vi "PIM Stimulus Key Array.vi"(4 "Conversion":enum16{"Cluster - HTML", "HTML - Cluster"}(ring), 6 "PIM Test Parameters":T1={"Stimulus"={"C1 Pwr dBm"=0.0, "C2 Pwr dBm"=0.0, "Power Units"=enum."dBm", "Meas Type"=enum."Time", "C1 Freq MHz"=0.0, "C2 Freq MHz"=0.0, "Swept Freq Step"=0}, "Measure"={"IM Order"=0, "Direction"=0, "Averaging"=1, "ALC ON?"=TRUE, "Peak Hold?"=TRUE, "Peak last N"=1, "Ref Level dBm"=-100.0, "Ref Units"=enum."dBm", "Num Samples"=1, "Sample units"=enum."Sample(s)", "Update Rate (s)"=0.0, "DUT PORT"=enum."Port 1", "Percent (%)"=100}, "Display"={"Power Scale"={"yRange_min"=0, "yRange_max"=0}, "xRange_span"=5}} {"Stimulus"."Swept Freq Step" items=[".2", ".4", "1.0", "2.0"]; "Measure"."Averaging" items=["None", "Minimum", "Normal", "High", "Maximum"]; "Measure"."Direction" items=["Reverse", "Forward", "Auxiliary"]; "Measure"."IM Order" items=["3rd", "5th", "7th", "9th", "11th", "13th", "15th", "17th", "19th", "21st", "23rd", "25th", "27th", "29th", "31st", "33rd"]}, 7 "Key Array In":T11) -> (1 "PIM Test Parameters (out)":T1={"Stimulus"={"C1 Pwr dBm"=0.0, "C2 Pwr dBm"=0.0, "Power Units"=enum."dBm", "Meas Type"=enum."Time", "C1 Freq MHz"=0.0, "C2 Freq MHz"=0.0, "Swept Freq Step"=0}, "Measure"={"IM Order"=0, "Direction"=0, "Averaging"=1, "ALC ON?"=TRUE, "Peak Hold?"=TRUE, "Peak last N"=1, "Ref Level dBm"=-100.0, "Ref Units"=enum."dBm", "Num Samples"=1, "Sample units"=enum."Sample(s)", "Update Rate (s)"=0.0, "DUT PORT"=enum."Port 1", "Percent (%)"=100}, "Display"={"Power Scale"={"yRange_min"=0, "yRange_max"=0}, "xRange_span"=5}} {"Stimulus"."Swept Freq Step" items=[".2", ".4", "1.0", "2.0"]; "Measure"."Averaging" items=["None", "Minimum", "Normal", "High", "Maximum"]; "Measure"."Direction" items=["Reverse", "Forward", "Auxiliary"]; "Measure"."IM Order" items=["3rd", "5th", "7th", "9th", "11th", "13th", "15th", "17th", "19th", "21st", "23rd", "25th", "27th", "29th", "31st", "33rd"]}, 2 "Key Array Out":T11)   [LabVIEW 2011]
uses:
  ITK/utils/keyedarr.llb/Keyed Array.ctl
  TypeDefs/PIM Test Parameters.ctl
  TypeDefs/PIM Stimulus Parameters.ctl
  BPIMCore/HW IO/PIM Sweep Step Size.ctl
  TypeDefs/PIM Measurement Parameters.ctl
  BPIMCore/HW IO/IMOrder.ctl
  BPIMCore/HW IO/MeasMode.ctl
  BPIMCore/HW IO/HW Averaging.ctl
  TypeDefs/PIM Meas Units.ctl
  BPIMCore/HW IO/DUTport.ctl
  TypeDefs/PIM Display Parameters.ctl
  ITK/utils/strutil.llb/Case Matching.ctl
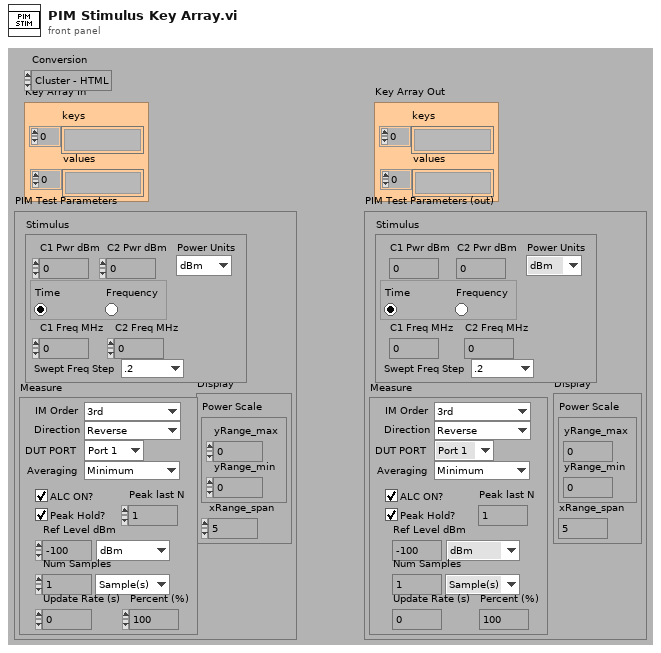
[diagram p1: front panel]
types:
  T1 = typedef "PIM Test Parameters.ctl" = cluster{"Stimulus":T2, "Measure":T4, "Display":T10}
  T2 = typedef "PIM Stimulus Parameters.ctl" = cluster{"C1 Pwr dBm":dbl, "C2 Pwr dBm":dbl, "Power Units":enum16{"dBm", "Watts"}, "Meas Type":enum32{"Time", "Frequency"}, "C1 Freq MHz":dbl, "C2 Freq MHz":dbl, "Swept Freq Step":T3}
  T3 = typedef "PIM Sweep Step Size.ctl" = u16
  T4 = typedef "PIM Measurement Parameters.ctl" = cluster{"IM Order":T5, "Direction":T6, "Averaging":T7, "ALC ON?":bool, "Peak Hold?":bool, "Peak last N":u32, "Ref Level dBm":dbl, "Ref Units":enum16{"dBm", "dBc"}, "Num Samples":u32, "Sample units":T8, "Update Rate (s)":dbl, "DUT PORT":T9, "Percent (%)":u8}
  T5 = typedef "IMOrder.ctl" = u8
  T6 = typedef "MeasMode.ctl" = u16
  T7 = typedef "HW Averaging.ctl" = u16
  T8 = typedef "PIM Meas Units.ctl" = enum16{"Sample(s)", "Second(s)", "Sweep(s)"}
  T9 = typedef "DUTport.ctl" = enum16{"Port 1", "Port 2"}
  T10 = typedef "PIM Display Parameters.ctl" = cluster{"Power Scale":cluster{"yRange_min":i32, "yRange_max":i32}, "xRange_span":u32}
  T11 = typedef "Keyed Array.ctl" = cluster{"keys":string[], "values":string[]}
  T12 = typedef "Case Matching.ctl" = enum16{"a != A", "a == A", "system"}
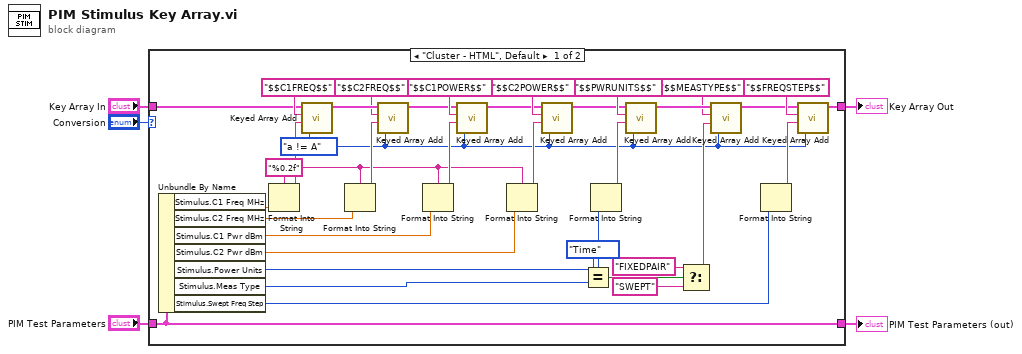
[diagram p0: block diagram]
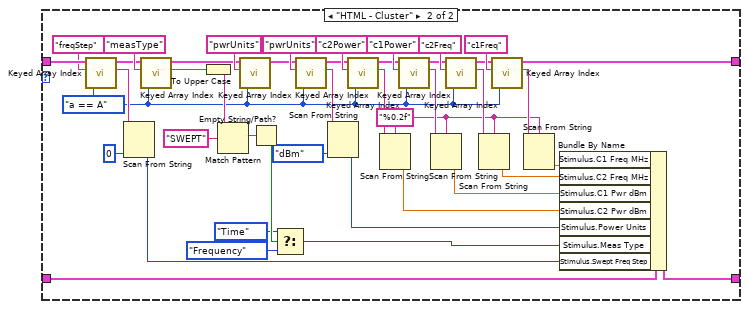
[diagram p2: hidden frame]
diagram:
  n1 = case shown="\"Cluster - HTML\", Default" "Conversion" {
    tunnel: "Key Array In" -> [w38 w84]
    tunnel: "PIM Test Parameters" -> [w9 w82]
    tunnel: [w27 w46] -> w3
    tunnel: [w9 w81] -> w2
    frame "Cluster - HTML", Default {
      w7 = "%0.2f" ("format string")
      w6 = Case_Matching."a != A" ("case matching (sensitive)")
      n2 = Unbundle By Name(w9) -> ("Stimulus.C1 Freq MHz"=w26:dbl, "Stimulus.C2 Freq MHz"=w24:dbl, "Stimulus.C1 Pwr dBm"=w22:dbl, "Stimulus.C2 Pwr dBm"=w19:dbl, "Stimulus.Power Units"=w18:enum16{"dBm", "Watts"}, "Stimulus.Meas Type"=w16:enum32{"Time", "Frequency"}, "Stimulus.Swept Freq Step"=w11:T3)
      n3 = Format Into String(format string=w7, w26) -> (resulting string=w25:string)  [unwired: 2 in, 1 out]
      n4 = call "Keyed Array Add.vi"("case matching (sensitive)"=w6, "value"=w25, "key"="$$C1FREQ$$", "array in"=w38) -> ("array out"=w41:T11)  [unwired: 3 out]
      n5 = Format Into String(format string=w7, w24) -> (resulting string=w23:string)  [unwired: 2 in, 1 out]
      n6 = call "Keyed Array Add.vi"("case matching (sensitive)"=w6, "value"=w23, "key"="$$C2FREQ$$", "array in"=w41) -> ("array out"=w34:T11)  [unwired: 3 out]
      n7 = Format Into String(format string=w7, w22) -> (resulting string=w21:string)  [unwired: 2 in, 1 out]
      n8 = call "Keyed Array Add.vi"("case matching (sensitive)"=w6, "value"=w21, "key"="$$C1POWER$$", "array in"=w34) -> ("array out"=w36:T11)  [unwired: 3 out]
      n9 = Format Into String(format string=w7, w19) -> (resulting string=w20:string)  [unwired: 2 in, 1 out]
      n10 = call "Keyed Array Add.vi"("case matching (sensitive)"=w6, "value"=w20, "key"="$$C2POWER$$", "array in"=w36) -> ("array out"=w28:T11)  [unwired: 3 out]
      n11 = Equal?(x=enum32{"Time", "Frequency"}."Time" ("Stimulus.Meas Type"), y=w16) -> (x = y?=w15:bool)
      n12 = Format Into String(w18) -> (resulting string=w17:string)  [unwired: 3 in, 1 out]
      n13 = call "Keyed Array Add.vi"("case matching (sensitive)"=w6, "value"=w17, "key"="$$PWRUNITS$$", "array in"=w28) -> ("array out"=w32:T11)  [unwired: 3 out]
      n14 = Select(t="FIXEDPAIR", s=w15, f="SWEPT") -> (s? t:f=w12:string)
      n15 = call "Keyed Array Add.vi"("case matching (sensitive)"=w6, "value"=w12, "key"="$$MEASTYPE$$", "array in"=w32) -> ("array out"=w29:T11)  [unwired: 3 out]
      n16 = Format Into String(w11) -> (resulting string=w10:string)  [unwired: 3 in, 1 out]
      n17 = call "Keyed Array Add.vi"("case matching (sensitive)"=w6, "value"=w10, "key"="$$FREQSTEP$$", "array in"=w29) -> ("array out"=w27:T11)  [unwired: 3 out]
    }
    frame "HTML - Cluster" {
      w42 = "%0.2f" ("format string")
      w43 = Case_Matching."a == A" ("case matching (sensitive)")
      n18 = call "Keyed Array Index.vi"("case matching (sensitive)"=w43, "key"="freqStep", "array in"=w84) -> ("value"=w49:string, "duplicate array"=w48:T11)  [unwired: 1 in, 2 out]
      n19 = Scan From String(input string=w49, default 1=0) -> (output 1=w47:i32)  [unwired: 3 in, 3 out]
      n20 = call "Keyed Array Index.vi"("case matching (sensitive)"=w43, "key"="measType", "array in"=w48) -> ("value"=w55:string, "duplicate array"=w57:T11)  [unwired: 1 in, 2 out]
      n21 = To Upper Case(1:w55) -> (0:w54:string)
      n22 = Match Pattern(string=w54, regular expression="SWEPT") -> (match substring=w53:string)  [unwired: 4 out]
      n23 = call "Keyed Array Index.vi"("case matching (sensitive)"=w43, "key"="pwrUnits", "array in"=w57) -> ("duplicate array"=w59:T11)  [unwired: 1 in, 3 out]
      n24 = Empty String/Path?(string/path=w53) -> (empty?=w52:bool)
      n25 = Select(t=enum32{"Time", "Frequency"}."Time" ("Stimulus.Meas Type"), s=w52, f=enum32{"Time", "Frequency"}."Frequency" ("Stimulus.Meas Type")) -> (s? t:f=w51:enum32{"Time", "Frequency"})
      n26 = call "Keyed Array Index.vi"("case matching (sensitive)"=w43, "key"="pwrUnits", "array in"=w59) -> ("value"=w62:string, "duplicate array"=w64:T11)  [unwired: 1 in, 2 out]
      n27 = Scan From String(input string=w62, default 1=enum16{"dBm", "Watts"}."dBm" ("Stimulus.Power Units")) -> (output 1=w61:enum16{"dBm", "Watts"})  [unwired: 3 in, 3 out]
      n28 = call "Keyed Array Index.vi"("case matching (sensitive)"=w43, "key"="c2Power", "array in"=w64) -> ("value"=w69:string, "duplicate array"=w67:T11)  [unwired: 1 in, 2 out]
      n29 = Scan From String(format string=w42, input string=w69) -> (output 1=w66:dbl)  [unwired: 2 in, 4 out]
      n30 = call "Keyed Array Index.vi"("case matching (sensitive)"=w43, "key"="c1Power", "array in"=w67) -> ("value"=w71:string, "duplicate array"=w72:T11)  [unwired: 1 in, 2 out]
      n31 = Scan From String(format string=w42, input string=w71) -> (output 1=w70:dbl)  [unwired: 2 in, 4 out]
      n32 = call "Keyed Array Index.vi"("case matching (sensitive)"=w43, "key"="c2Freq", "array in"=w72) -> ("value"=w75:string, "duplicate array"=w76:T11)  [unwired: 1 in, 2 out]
      n33 = Scan From String(format string=w42, input string=w75) -> (output 1=w74:dbl)  [unwired: 2 in, 4 out]
      n34 = call "Keyed Array Index.vi"("case matching (sensitive)"=w43, "key"="c1Freq", "array in"=w76) -> ("value"=w79:string, "duplicate array"=w46:T11)  [unwired: 1 in, 2 out]
      n35 = Scan From String(format string=w42, input string=w79) -> (output 1=w80:dbl)  [unwired: 2 in, 4 out]
      n36 = Bundle By Name(cluster=w82, "Stimulus.C1 Freq MHz"=w80, "Stimulus.C2 Freq MHz"=w74, "Stimulus.C1 Pwr dBm"=w70, "Stimulus.C2 Pwr dBm"=w66, "Stimulus.Power Units"=w61, "Stimulus.Meas Type"=w51, "Stimulus.Swept Freq Step"=w47) -> (w81:T1)
    }
  }
  "Key Array Out" <- w3
  "PIM Test Parameters (out)" <- w2
